vi "generate event.vi"(10 "event":T1, 11 "event queue in":T2) -> (1 "failed?":bool, 3 "event queue out":T2)   [LabVIEW 2013, in "data bus events.lvlib"]
uses:
  data bus events.lvlib
  event queue.ctl
  event.ctl
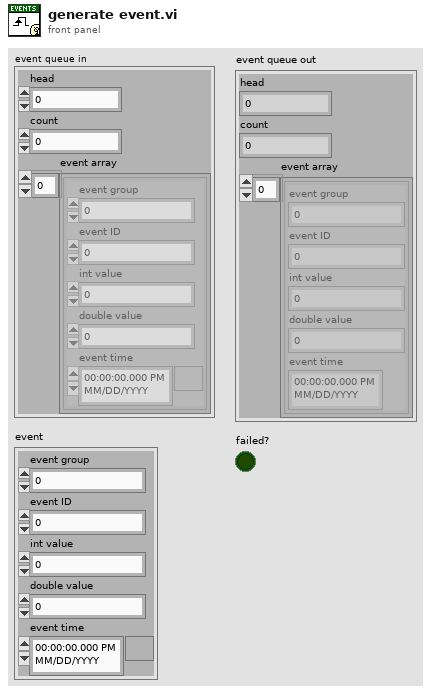
[diagram p1: front panel]
types:
  T1 = typedef "data bus events.lvlib/event.ctl" = cluster{"event group":i64, "event ID":i64, "int value":i64, "double value":dbl, "event time":timestamp}
  T2 = typedef "data bus events.lvlib/event queue.ctl" = cluster{"head":i32, "count":i32, "event array":T1[]}
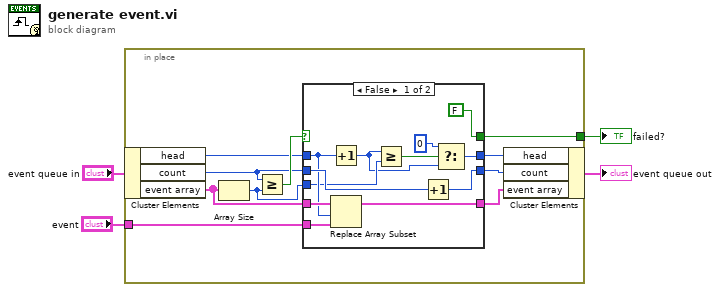
[diagram p0: block diagram]
diagram:
  n1 = in-place {
    in-place-border: "event" -> [w13]
    in-place-border: [w12] -> w3
    n2 = in-place-cluster #1("event queue in") -> ("head"=w7:i32, "count"=w10:i32, "event array"=w11:T1[])
    n3 = Array Size(array=w11) -> (size(s)=w6:i32)
    n4 = Greater Or Equal?(x=w10, y=w6) -> (x >= y?=w14:bool)
    n5 = case shown="False" w14 {
      selector: w14 -> [_ w30]
      tunnel: w13 -> [w23 _]
      tunnel: [FALSE w30] -> w12
      tunnel: w11 -> [w25 w28]
      tunnel: w10 -> [w22 w29]
      tunnel: [w21 w29] -> w9
      tunnel: [w24 w28] -> w8
      tunnel: w7 -> [w20 w27]
      tunnel: w6 -> [w18 _]
      tunnel: [w16 w27] -> w5
      frame False {
        n6 = Increment(x=w20) -> (x+1=w17:i32)
        n7 = Replace Array Subset(array=w25, new element=w23, index=w20) -> (w24:T1[])
        n8 = Greater Or Equal?(x=w17, y=w18) -> (x >= y?=w19:bool)
        n9 = Increment(x=w22) -> (x+1=w21:i32)
        n10 = Select(t=0, s=w19, f=w17) -> (s? t:f=w16:i32)
      }
      frame True {
      }
    }
    n11 = in-place-cluster #1("head"=w5, "count"=w9, "event array"=w8) -> (→"event queue out":T2)
  }
  "failed?" <- w3
